vi "example - Test Client.vi"() -> ()   [LabVIEW 2019, in "Service.lvlib"]
uses:
  Service.lvlib
  mmw_command_lib/src_LabVIEW/mmW_commands/TypeDefs/cmd_list.ctl
  SubVIs/Client-states.ctl
  SubVIs/ClientAppData.ctl
  <vilib>/addons/zeromq/zmq_socket.lvclass
  <vilib>/addons/zeromq/zmq_context.lvclass
  <vilib>/addons/zeromq/socket_type.ctl
  <vilib>/addons/zeromq/zeromq.lvlib
  mmw_command_lib/src_LabVIEW/mmW_commands/mmW_commands.lvlib
panel:
  out "parts":string[](array[string])
  out "Array":errorcluster[](array[cluster])
  out "error out":errorcluster
  out "Client-states":T1
  in  "?":T2
  in  "SendCmd":bool
  in  "stop":bool
  in  "endpoint":string="tcp://127.0.0.1:5555"
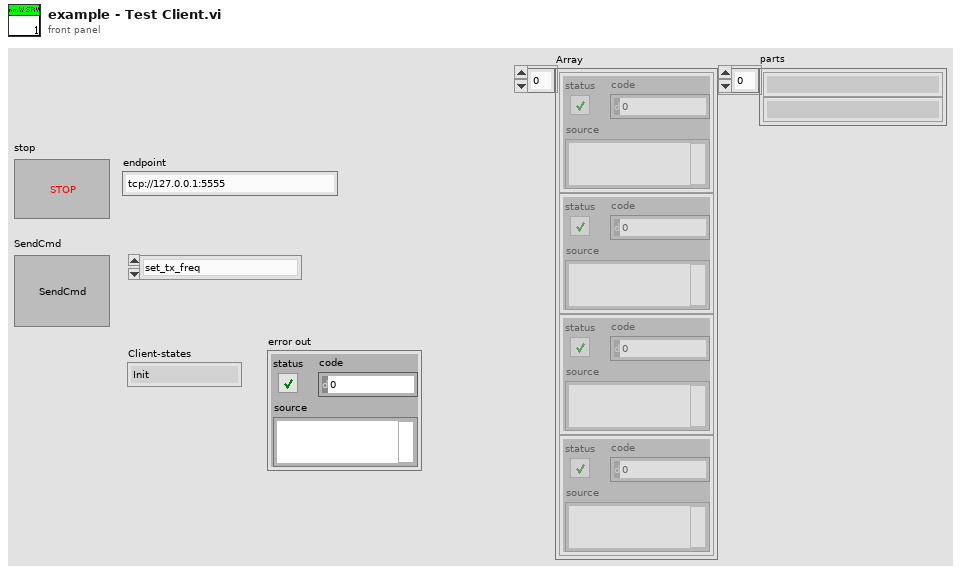
[diagram p1: front panel]
types:
  T1 = typedef "Service.lvlib/Client-states.ctl" = enum16{"Init", "Idle", "SendCmd", "ReceiveResp", "Shutdown"}
  T2 = typedef "mmW_commands.lvlib/cmd_list.ctl" = enum16{"set_tx_freq", "store_waveform", "free_message"}
  T3 = typedef "Service.lvlib/ClientAppData.ctl" = cluster{"ZMQ":cluster{"socket ":refnum<class "zmq_socket.lvclass">, "context":refnum<class "zmq_context.lvclass">}}
  T4 = typedef "zeromq.lvlib/socket_type.ctl" = enum8{"ZMQ_PAIR", "ZMQ_PUB", "ZMQ_SUB", "ZMQ_REQ", "ZMQ_REP", "ZMQ_DEALER", "ZMQ_ROUTER", "ZMQ_PULL", "ZMQ_PUSH", "ZMQ_XPUB", "ZMQ_XSUB"}
  T5 = cluster{"socket ":refnum<class "zmq_socket.lvclass">, "context":refnum<class "zmq_context.lvclass">}
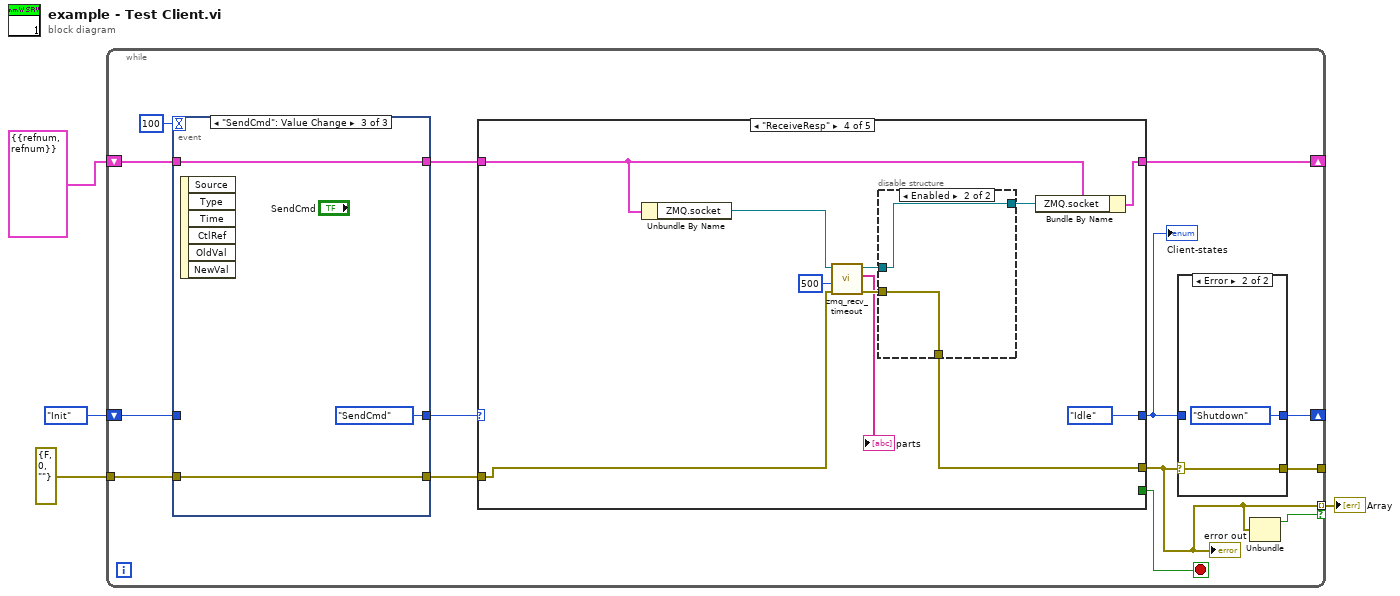
[diagram p0: block diagram]
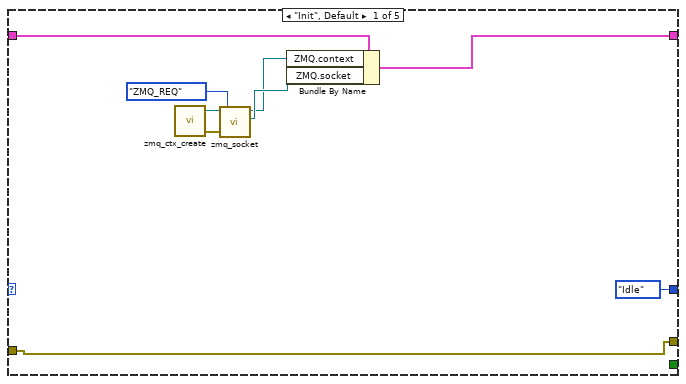
[diagram p3: hidden frame]
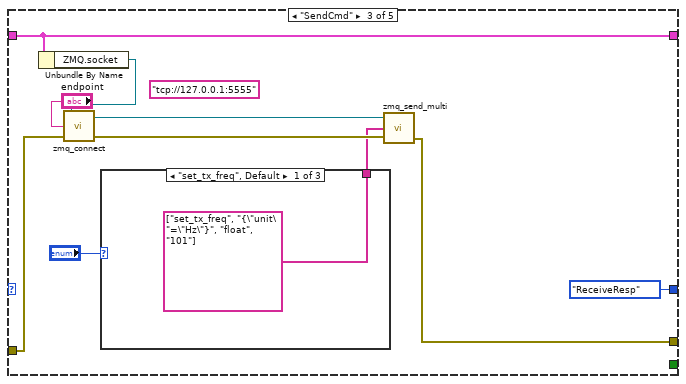
[diagram p5: hidden frame]
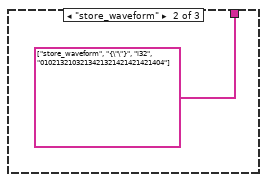
[diagram p6: hidden frame]
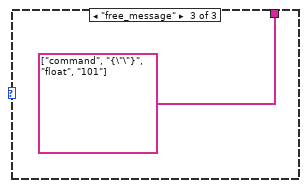
[diagram p7: hidden frame]
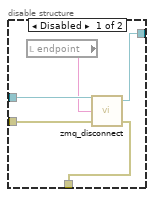
[diagram p8: hidden frame]
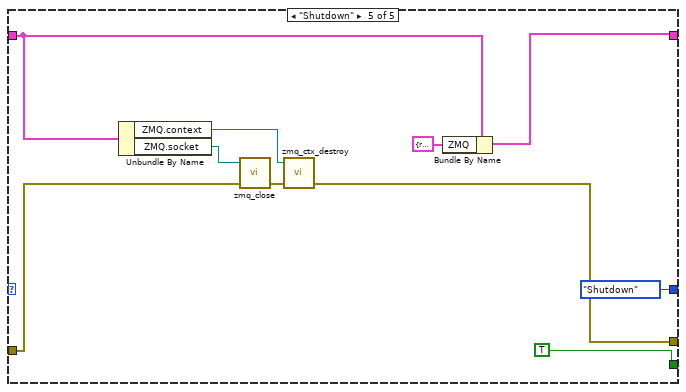
[diagram p9: hidden frame]
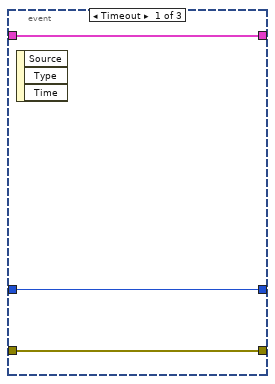
[diagram p10: hidden frame]
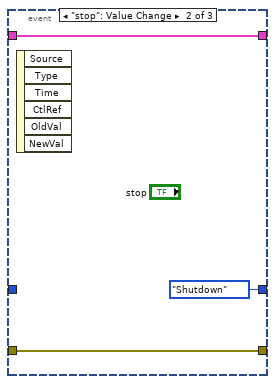
[diagram p11: hidden frame]
diagram:
  n1 = while {
    shift-right: [w7] -> _
    shift-left: Client-states."Init" -> [w18]
    shift-right: [w13] -> _
    shift-left: T3 {"ZMQ"={"socket "=refnum, "context"=refnum}} -> [w15]
    tunnel: errorcluster {"status"=FALSE, "code"=0, "source"=""} ("error constant") -> [w12]
    tunnel: [w9] -> _
    tunnel: [w6] -> w1 mode=indexing if=w5
    stop <- w10 stop-if-true
    n2 = event shown="[2] \"SendCmd\": Value Change" {
      selector: _ -> [_ _ _]
      dyn-events: _ -> [_ _ _]
      timeout: 100 -> [_ _ _]
      tunnel: w18 -> [w78 _ _]
      tunnel: [w78 Client-states."Shutdown" Client-states."SendCmd"] -> w17
      tunnel: w15 -> [w77 w80 w84]
      tunnel: [w77 w80 w84] -> w14
      tunnel: w12 -> [w76 w79 w82]
      tunnel: [w76 w79 w82] -> w11
      event Timeout {
        n3 = event-data() -> ()  [unwired: 1 in, 3 out]
      }
      event "stop": Value Change {
        n4 = event-data() -> ()  [unwired: 1 in, 6 out]
      }
      event "SendCmd": Value Change {
        n5 = event-data() -> ()  [unwired: 1 in, 6 out]
      }
    }
    n6 = case shown="\"ReceiveResp\"" w17 {
      selector: w17 -> [_ w32 _ _ _]
      tunnel: w14 -> [w28 w34 w43 w52 w73]
      tunnel: [w25 w34 w43 w50 w71] -> w13
      tunnel: w11 -> [w24 w33 w40 w56 w67]
      tunnel: [w24 w33 w39 w54 w74] -> w6
      tunnel: [Client-states."Idle" ("Client-states") w32 Client-states."ReceiveResp" Client-states."Idle" ("Client-states") Client-states."Shutdown" ("Client-states")] -> w8
      tunnel: [_ _ _ _ TRUE] -> w10
      frame "Init", Default {
        n7 = call <vilib>:"zmq_ctx_create.vi"() -> ("error out"=w30:errorcluster, "context out"=w31:refnum<class "zmq_context.lvclass">)  [unwired: 4 in]
        n8 = call <vilib>:"zmq_socket.vi"("error in"=w30, "socket type"=socket_type."ZMQ_REQ", "context in"=w31) -> ("socket out"=w27:refnum<class "zmq_socket.lvclass">, "context out"=w26:refnum<class "zmq_context.lvclass">)  [unwired: 2 in, 1 out]
        n9 = Bundle By Name(cluster=w28, "ZMQ.context"=w26, "ZMQ.socket"=w27) -> (w25:T3)
      }
      frame "Idle" {
      }
      frame "SendCmd" {
        (unwired) "tcp://127.0.0.1:5555" ("endpoint")
        n10 = Unbundle By Name(w43) -> ("ZMQ.socket"=w42:refnum<class "zmq_socket.lvclass">)
        n11 = call <vilib>:"zmq_connect.vi"("error in"=w40, "endpoint"="endpoint", "socket in"=w42) -> ("error out"=w41:errorcluster, "socket out"=w38:refnum<class "zmq_socket.lvclass">)  [unwired: 1 in]
        n12 = case shown="\"set_tx_freq\", Default" "?" {
          tunnel: [string[] ["set_tx_freq", "{\"unit\"=\"Hz\"}", "float", "101"] string[] ["store_waveform", "{\"\"}", "i32", "0102132103213421321421421421404"] string[] ["command", "{\"\"}", "float", "101"]] -> w35
          frame "set_tx_freq", Default {
          }
          frame "store_waveform" {
          }
          frame "free_message" {
          }
        }
        n13 = call <vilib>:"zmq_send_multi.vi"("error in"=w41, "parts"=w35, "socket in"=w38) -> ("error out"=w39:errorcluster)  [unwired: 1 in, 1 out]
      }
      frame "ReceiveResp" {
        n14 = Unbundle By Name(w52) -> ("ZMQ.socket"=w57:refnum<class "zmq_socket.lvclass">)
        n15 = call <vilib>:"zmq_recv_timeout.vi"("error in"=w56, "timeout (ms)"=u32 500, "socket in"=w57) -> ("error out"=w55:errorcluster, "parts"=→"parts":string[], "socket out"=w53:refnum<class "zmq_socket.lvclass">)  [unwired: 1 in, 1 out]
        n16 = disable-structure shown="Enabled" {
          disable-tunnel: w55 -> [w63 w65]
          disable-tunnel: [w62 w65] -> w54
          disable-tunnel: w53 -> [w61 w64]
          disable-tunnel: [w59 w64] -> w51
          frame Disabled {
            n17 = local read "endpoint"() -> (w60:string)
            n18 = call <vilib>:"zmq_disconnect.vi"("error in"=w63, "endpoint"=w60, "socket in"=w61) -> ("error out"=w62:errorcluster, "socket out"=w59:refnum<class "zmq_socket.lvclass">)  [unwired: 1 in]
          }
          frame Enabled {
          }
        }
        n19 = Bundle By Name(cluster=w52, "ZMQ.socket"=w51) -> (w50:T3)
      }
      frame "Shutdown" {
        n20 = Unbundle By Name(w73) -> ("ZMQ.context"=w75:refnum<class "zmq_context.lvclass">, "ZMQ.socket"=w68:refnum<class "zmq_socket.lvclass">)
        n21 = call <vilib>:"zmq_close.vi"("error in"=w67, "socket"=w68) -> ("error out"=w66:errorcluster)  [unwired: 3 in]
        n22 = call <vilib>:"zmq_ctx_destroy.vi"("error in"=w66, "context in"=w75) -> ("error out"=w74:errorcluster)  [unwired: 3 in]
        n23 = Bundle By Name(cluster=w73, "ZMQ"=T5 {"socket "=refnum, "context"=refnum}) -> (w71:T3)
      }
    }
    "Client-states" <- w8
    "error out" <- w6
    n24 = case shown="Error" w6 {
      selector: w6 -> [w20 w22]
      tunnel: [w20 w22] -> w9
      tunnel: w8 -> [w19 _]
      tunnel: [w19 Client-states."Shutdown" ("Client-states")] -> w7
      frame No Error {
      }
      frame Error {
      }
    }
    n25 = Unbundle(w6) -> ("status"=w5:bool)  [unwired: 2 out]
  }
  "Array" <- w1
